vi "Send VI Panel Reference to Caller.vi"(8 "error in (no error)":errorcluster, 11 "Grid Screen in":refnum<class "Grid Screen.lvclass">) -> (0 "error out":errorcluster, 3 "Grid Screen out":refnum<class "Grid Screen.lvclass">)   [LabVIEW 2024, in "Grid Screen.lvlib" / "Grid Screen.lvclass"]
uses:
  Grid Screen.lvclass
  Applications/National Instruments/LabVIEW 2024 64-bit/vi.lib/ActorFramework/Actor/Actor.lvclass
  <vilib>/ActorFramework/Actor/Actor.lvclass/Actor.ctl
  Grid Screen.lvclass/Grid Screen.ctl
  Controller/Controller Messages/Load Main Panel Display Msg/Load Main Panel Display Msg.lvclass/Load Main Panel Display Msg.ctl
  <vilib>/ActorFramework/Message Enqueuer/Message Enqueuer.lvclass/Message Enqueuer.ctl
  <vilib>/ActorFramework/Message Enqueuer/Enqueue.vi
  Controller/Controller Messages/Load Main Panel Display Msg/Load Main Panel Display Msg.lvclass
  Applications/National Instruments/LabVIEW 2024 64-bit/vi.lib/ActorFramework/Message/Message.lvclass
  <vilib>/ActorFramework/Message Priority Queue/Priority Enqueue.vi
  <vilib>/ActorFramework/Actor/Actor.lvclass
  Controller/Controller Messages/Write Grid Panel Reference Msg/Write Grid Panel Reference Msg.lvclass
  Users/elijahkerry/challenge-of-champions/MC Screen/MC Screen/Grid Screen.lvclass
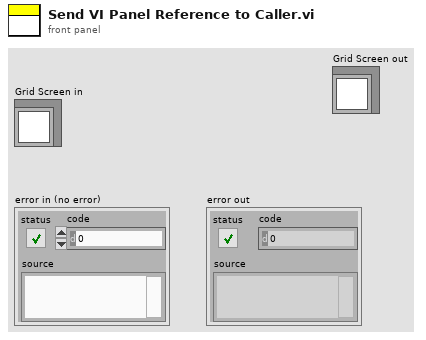
[diagram p1: front panel]
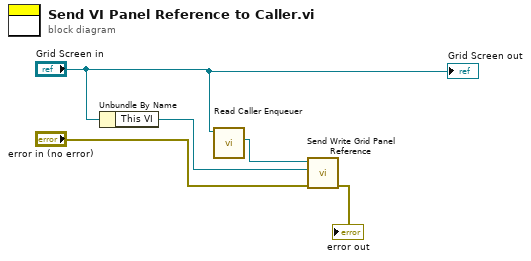
[diagram p0: block diagram]
diagram:
  n1 = Unbundle By Name("Grid Screen in") -> ("This VI"=w3:refnum<vi>)
  n2 = call <vilib>:"Read Caller Enqueuer.vi"("Actor"="Grid Screen in") -> ("Caller Enqueuer"=w4:refnum<class "Message Enqueuer.lvclass">)  [unwired: 10 in]
  n3 = call "Send Write Grid Panel Reference.vi"("error in (no error)"="error in (no error)", "Grid Panel Reference"=w3, "Message Enqueuer"=w4) -> ("error out"=→"error out":errorcluster)  [unwired: 7 in, 1 out]
  "Grid Screen out" <- "Grid Screen in"
